vi "PT3_Create.vi"(4 "Image Header in":T2, 5 "Save pt3":bool=TRUE, 6 "Measurement Type":T1(ring)=enum."Point Measurement", 7 "overwrite existing":bool, 8 "error in":errorcluster, 9 "Comment":string, 10 "pt3 Header in":T3={"Comment"="", "RangeNo"=0, "Offset"=0, "AcquisitionTime (ms)"=0, "HardwareSerial"=0, "SyncDivider"=0, "Resolution (ns)"=0.0, "CFD Settings"={"Ch0 Level"=150, "Ch0 ZeroX"=10, "Ch1 Level"=50, "Ch1 ZeroX"=10}, "InpRate0"=0, "InpRate1"=0}, 11 "File Path":path) -> (0 "error out":errorcluster, 3 "refnum out":refnum<file>)   [LabVIEW 2010]
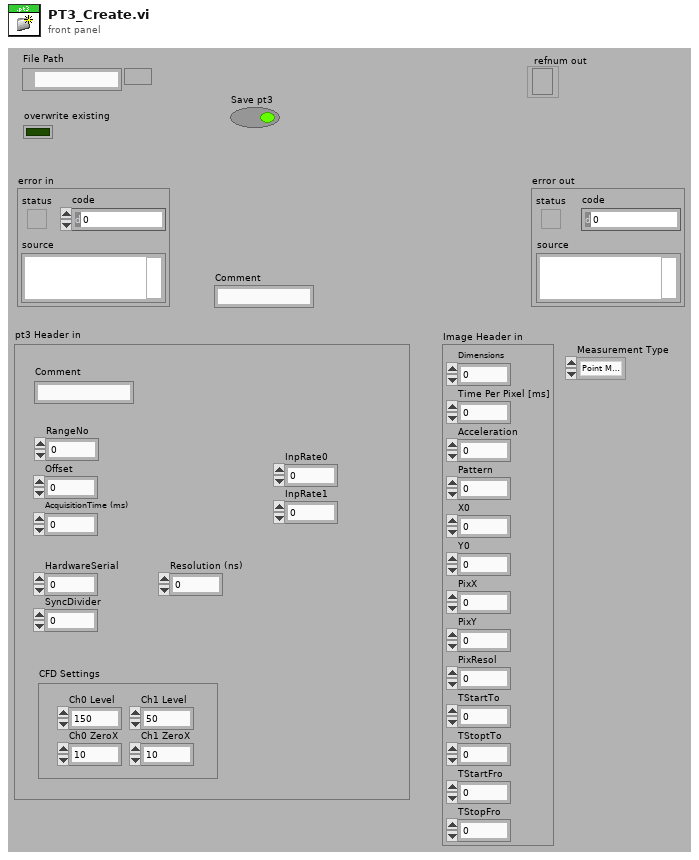
[diagram p1: front panel]
types:
  T1 = enum16{"not a pt3 File", "Image File", "Point Measurement", "Auto Point"}
  T2 = cluster{"Dimensions":i32, "Time Per Pixel [ms]":dbl, "Acceleration":i32, "Pattern":i32, "X0":sgl, "Y0":sgl, "PixX":i32, "PixY":i32, "PixResol":sgl, "TStartTo":sgl, "TStoptTo":sgl, "TStartFro":sgl, "TStopFro":sgl}
  T3 = cluster{"Comment":string, "RangeNo":i32, "Offset":i32, "AcquisitionTime (ms)":i32, "HardwareSerial":i32, "SyncDivider":i32, "Resolution (ns)":sgl, "CFD Settings":cluster{"Ch0 Level":i32, "Ch0 ZeroX":i32, "Ch1 Level":i32, "Ch1 ZeroX":i32}, "InpRate0":i32, "InpRate1":i32}
  T4 = enum16{"big-endian, network order", "native, host order", "little-endian"}
  T5 = enum16{"open", "replace", "create", "open or create", "replace or create", "replace or create with confirmation"}
  T6 = cluster{"HardwareSerial":i32, "SyncDivider":i32, "Ch0 ZeroX":i32, "Ch0 Level":i32, "Ch1 ZeroX":i32, "Ch1 Level":i32, "Resolution (ns)":sgl, "RouterModelCode":i32, "RouterEnabled":i32}
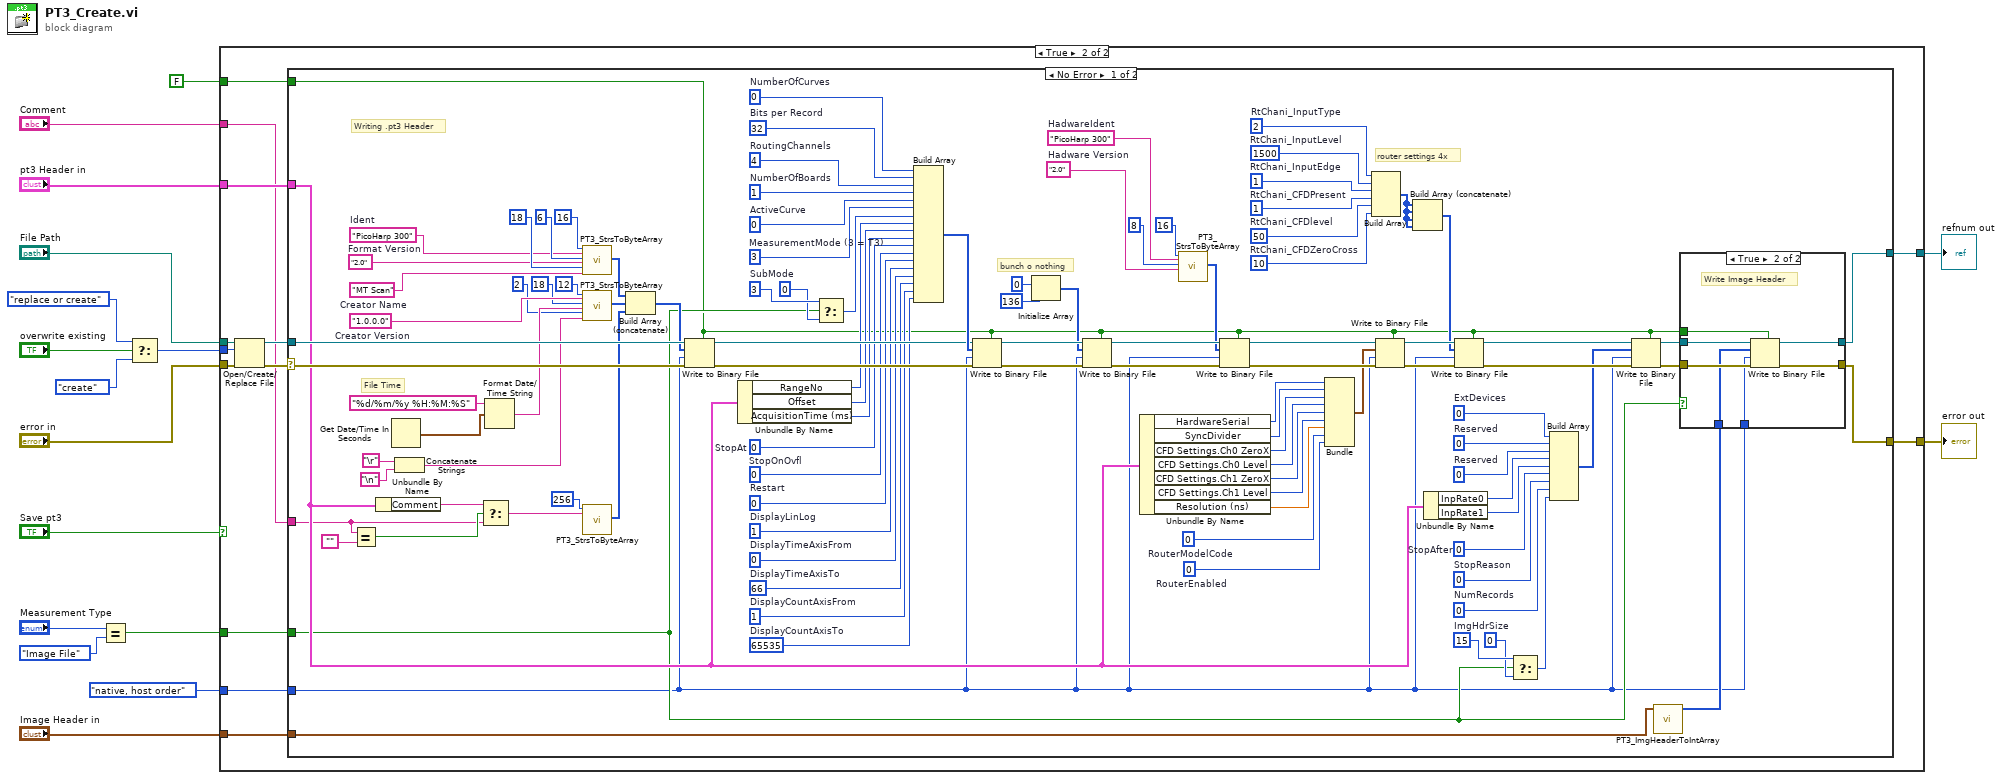
[diagram p0: block diagram]
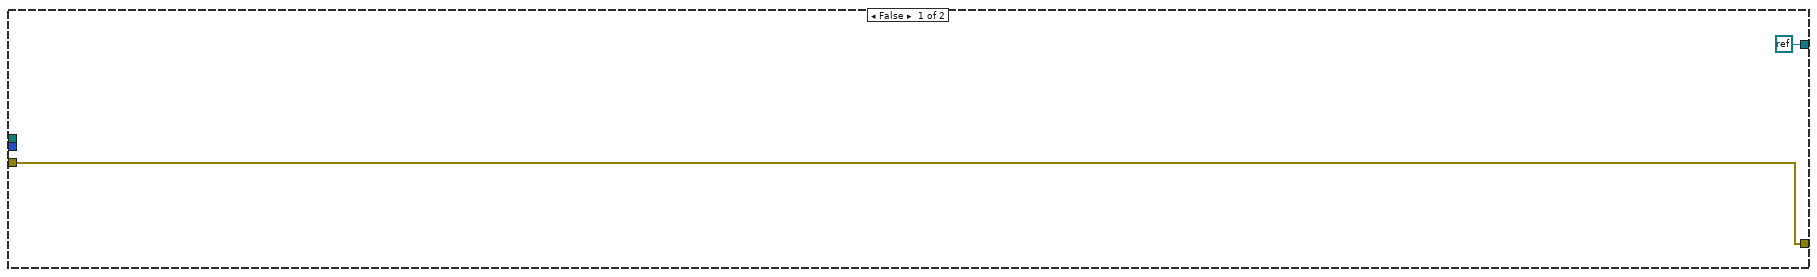
[diagram p2: hidden frame]
diagram:
  n1 = Equal?(x="Measurement Type", y=T1."Image File") -> (x = y?=w2:bool)
  n2 = Select(t=T5."replace or create" ("operation (0:open)"), s="overwrite existing", f=T5."create" ("operation (0:open)")) -> (s? t:f=w13:T5)
  n3 = case shown="True" "Save pt3" {
    tunnel: "File Path" -> [_ w32]
    tunnel: w13 -> [_ w31]
    tunnel: "error in" -> [w19 w30]
    tunnel: [w19 w28] -> w11
    tunnel: [refnum<k0> refnum w26] -> w10
    tunnel: "pt3 Header in" -> [_ w25]
    tunnel: T4."native, host order" ("byte order (0:big-endian, network order)") -> [_ w24]
    tunnel: FALSE ("prepend array or string size? (T)") -> [_ w23]
    tunnel: "Comment" -> [_ w22]
    tunnel: w2 -> [_ w21]
    tunnel: "Image Header in" -> [_ w20]
    frame False {
    }
    frame True {
      n4 = Open/Create/Replace File(file path (use dialog)=w32, error in=w30, operation (0:open)=w31) -> (refnum out=w27:refnum<file>, error out=w29:errorcluster)  [unwired: 4 out]
      n5 = case shown="No Error" w29 {
        selector: w29 -> [w141 w152]
        tunnel: [w38 w152] -> w28
        tunnel: w27 -> [w140 w151]
        tunnel: [w36 w151] -> w26
        tunnel: w25 -> [w63 _]
        tunnel: w24 -> [w33 _]
        tunnel: w23 -> [w35 _]
        tunnel: w22 -> [w49 _]
        tunnel: w21 -> [w40 _]
        tunnel: w20 -> [w41 _]
        frame No Error {
          w44 = 15  # ImgHdrSize
          w55 = 0  # NumRecords
          w56 = 0  # StopReason
          w57 = 0  # StopAfter
          w60 = 0  # Reserved
          w61 = 0  # Reserved
          w62 = 0  # ExtDevices
          w68 = 10  # RtChani_CFDZeroCross
          w70 = 50  # RtChani_CFDlevel
          w69 = 1  # RtChani_CFDPresent
          w71 = 1  # RtChani_InputEdge
          w72 = 1500  # RtChani_InputLevel
          w73 = 2  # RtChani_InputType
          w78 = 0  # RouterModelCode
          w77 = 0  # RouterEnabled
          w88 = "2.0"  # Hadware Version
          w90 = "PicoHarp 300"  # HadwareIdent
          w99 = 65535  # DisplayCountAxisTo
          w100 = 1  # DisplayCountAxisFrom
          w101 = 66  # DisplayTimeAxisTo
          w102 = 0  # DisplayTimeAxisFrom
          w103 = 1  # DisplayLinLog
          w104 = 0  # Restart
          w105 = 0  # StopOnOvfl
          w106 = 0  # StopAt
          w47 = 3  # SubMode
          w110 = 3  # MeasurementMode (3 = T3)
          w111 = 0  # ActiveCurve
          w112 = 1  # NumberOfBoards
          w113 = 4  # RoutingChannels
          w116 = 32  # Bits per Record
          w117 = 0  # NumberOfCurves
          w129 = "1.0.0.0"  # Creator Version
          w130 = "MT Scan"  # Creator Name
          w131 = "2.0"  # Format Version
          w132 = "PicoHarp 300"  # Ident
          # "router settings 4x"
          # "bunch o nothing"
          # "File Time"
          # "Writing .pt3 Header"
          n6 = Equal?(x=w49, y="") -> (x = y?=w51:bool)
          n7 = Unbundle By Name(w63) -> ("Comment"=w50:string)
          n8 = Get Date/Time In Seconds() -> (seconds since 1Jan1904=w137:timestamp)
          n9 = Concatenate Strings("\r", "\n") -> (w127:string)
          n10 = Select(t=w50, s=w51, f=w49) -> (s? t:f=w48:string)
          n11 = Format Date/Time String(time format string (%c)="%d/%m/%y %H:%M:%S", seconds (now)=w137) -> (date/time string=w128:string)  [unwired: 1 out]
          n12 = call "PT3_StrsToByteArray.vi"("Length"=16, "String"=w132, "Length 2"=6 ("Length"), "String 2"=w131, "Length 3"=18 ("Length"), "String 3"=w130) -> ("Byte Array"=w123:u8[])  [unwired: 1 in, 12 out]
          n13 = call "PT3_StrsToByteArray.vi"("Length"=12, "String"=w129, "Length 2"=18 ("Length"), "String 2"=w128, "Length 3"=2 ("Length"), "String 3"=w127) -> ("Byte Array"=w122:u8[])  [unwired: 1 in, 12 out]
          n14 = call "PT3_StrsToByteArray.vi"("Length"=256, "String"=w48) -> ("Byte Array"=w120:u8[])  [unwired: 5 in, 12 out]
          n15 = Build Array (concatenate)(w123, w122, w120) -> (w119:u8[])
          n16 = Write to Binary File(file (use dialog)=w140, data=w119, error in=w141, 5:w35, 9:w33) -> (refnum out=w114:refnum<file>, error out=w115:errorcluster)  [unwired: 2 out]
          n17 = Unbundle By Name(w63) -> ("RangeNo"=w109:i32, "Offset"=w108:i32, "AcquisitionTime (ms)"=w107:i32)
          n18 = Select(t=w47, s=w40, f=0) -> (s? t:f=w45:i32)
          n19 = Build Array(w117, w116, w113, w112, w111, w110, w45, w109, w108, w107, w106, w105, w104, w103, w102, w101, w100, w99) -> (w118:i32[])
          n20 = Write to Binary File(file (use dialog)=w114, data=w118, error in=w115, 5:w35, 9:w33) -> (refnum out=w97:refnum<file>, error out=w98:errorcluster)  [unwired: 2 out]
          n21 = Initialize Array(u8 0 ("element"), 136 ("dimension size")) -> (w94:u8[])
          n22 = Write to Binary File(file (use dialog)=w97, data=w94, error in=w98, 5:w35, 9:w33) -> (refnum out=w92:refnum<file>, error out=w93:errorcluster)  [unwired: 2 out]
          n23 = Unbundle By Name(w63) -> ("HardwareSerial"=w84:i32, "SyncDivider"=w83:i32, "CFD Settings.Ch0 ZeroX"=w82:i32, "CFD Settings.Ch0 Level"=w81:i32, "CFD Settings.Ch1 ZeroX"=w80:i32, "CFD Settings.Ch1 Level"=w79:i32, "Resolution (ns)"=w53:sgl)
          n24 = call "PT3_StrsToByteArray.vi"("Length"=16, "String"=w90, "Length 2"=8, "String 2"=w88) -> ("Byte Array"=w91:u8[])  [unwired: 3 in, 12 out]
          n25 = Write to Binary File(file (use dialog)=w92, data=w91, error in=w93, 5:w35, 9:w33) -> (refnum out=w85:refnum<file>, error out=w86:errorcluster)  [unwired: 2 out]
          n26 = Bundle("HardwareSerial"=w84, "SyncDivider"=w83, "Ch0 ZeroX"=w82, "Ch0 Level"=w81, "Ch1 ZeroX"=w80, "Ch1 Level"=w79, "Resolution (ns)"=w53, "RouterModelCode"=w78, "RouterEnabled"=w77) -> (w76:T6)  [unwired: 1 out]
          n27 = Build Array(w73, w72, w71, w69, w70, w68) -> (w67:i32[])
          n28 = Write to Binary File(file (use dialog)=w85, data=w76, error in=w86, 5:w35, 9:w33) -> (refnum out=w74:refnum<file>, error out=w75:errorcluster)  [unwired: 2 out]
          n29 = Build Array (concatenate)(w67, w67, w67, w67) -> (w66:i32[])
          n30 = Unbundle By Name(w63) -> ("InpRate0"=w59:i32, "InpRate1"=w58:i32)
          n31 = Write to Binary File(file (use dialog)=w74, data=w66, error in=w75, 5:w35, 9:w33) -> (refnum out=w64:refnum<file>, error out=w65:errorcluster)  [unwired: 2 out]
          n32 = Select(t=w44, s=w40, f=0) -> (s? t:f=w43:i32)
          n33 = Build Array(w62, w61, w60, w59, w58, w57, w56, w55, w43) -> (w54:i32[])
          n34 = Write to Binary File(file (use dialog)=w64, data=w54, error in=w65, 5:w35, 9:w33) -> (refnum out=w37:refnum<file>, error out=w39:errorcluster)  [unwired: 2 out]
          n35 = call "PT3_ImgHeaderToIntArray.vi"("Image Header"=w41) -> ("Array"=w34:i32[])  [unwired: 10 out]
          n36 = case shown="True" w40 {
            tunnel: w39 -> [w142 w150]
            tunnel: [w142 w149] -> w38
            tunnel: w37 -> [w143 w148]
            tunnel: [w143 w147] -> w36
            tunnel: w35 -> [_ w146]
            tunnel: w34 -> [_ w145]
            tunnel: w33 -> [_ w144]
            frame False {
            }
            frame True {
              # "Write Image Header"
              n37 = Write to Binary File(file (use dialog)=w148, data=w145, error in=w150, 5:w146, 9:w144) -> (refnum out=w147:refnum<file>, error out=w149:errorcluster)  [unwired: 2 out]
            }
          }
        }
        frame Error {
        }
      }
    }
  }
  "refnum out" <- w10
  "error out" <- w11
